vi "Device.UnInit.vi"(8 "error in (no error)":errorcluster, 11 "SMU.Keithley2600":refnum<class "SMU.Keithley2600.lvclass">) -> (0 "error out":errorcluster, 3 "SMU.Keithley2600 out":refnum<class "SMU.Keithley2600.lvclass">)   [LabVIEW 2019, in "SMU.Keithley2600.lvclass"]
doc: "---------------------------------------------------------------\nJKI State Machine Objects™\nhttp://jki.net/state-machine-objects/\nCopyright (C) 2005-2015, JKI <info@jki.net>\nALL RIGHTS RESERVEDJKI State Machine Objects (SMO) 1.0.0.5\nJKI - JKI\nCopyright (c) 2016, JKI"
uses:
  SMU.Keithley2600.lvclass
  SMU/SMU.lvclass
  <instrlib>/Keithley 2600 Series/Keithley 2600 Series.lvlib
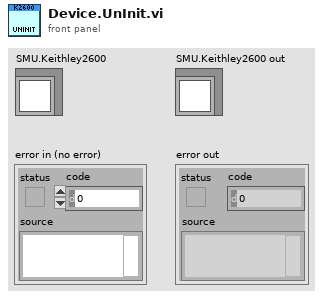
[diagram p1: front panel]
types:
  T1 = typedef "SMU.Keithley2600.lvclass/Resource--Cluster.ctl" = cluster{"VISA resource":refnum<visa-resource-name>, "Channel":i32}
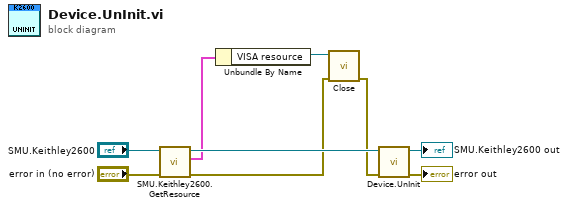
[diagram p0: block diagram]
diagram:
  n1 = call "SMU.Keithley2600.GetResource.vi"("error in (no error)"="error in (no error)", "SMU.Keithley2600 in"="SMU.Keithley2600") -> ("error out"=w5:errorcluster, "Resource"=w2:T1, "SMU.Keithley2600 out"=w6:refnum<class "SMU.Keithley2600.lvclass">)  [unwired: 7 in]
  n2 = Unbundle By Name(w2) -> ("VISA resource"=w1:refnum<visa-resource-name>)
  n3 = call <instrlib>:"Close.vi"("error in (no error)"=w5, "VISA resource name"=w1) -> ("error out"=w4:errorcluster)  [unwired: 9 out]
  n4 = call-parent "Device.UnInit.vi"("error in (no error)"=w4, "Device in"=w6) -> ("error out"=→"error out":errorcluster, "Device out"=→"SMU.Keithley2600 out":refnum<class "SMU.Keithley2600.lvclass">)  [unwired: 8 in]
